vi "user input.vi"(8 "error in":errorcluster) -> (0 "error out":errorcluster, 3 "Inputs from system":T1 {"Enabled" format="%.0x"})   [LabVIEW 2017, in "BuckBoost runtime.lvclass"]
uses:
  BuckBoost runtime.lvclass
  input user data.ctl
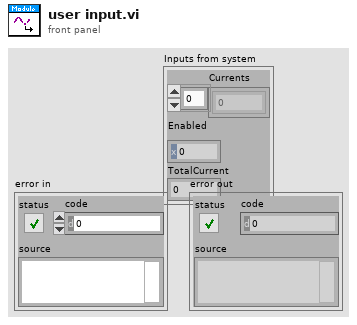
[diagram p1: front panel]
types:
  T1 = typedef "BuckBoost runtime.lvclass/input user data.ctl" = cluster{"Currents":dbl[], "Enabled":u8, "TotalCurrent":dbl}
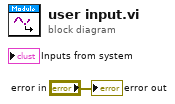
[diagram p0: block diagram]
diagram:
  "error out" <- "error in"
